vi "Arcade Drive.vi"(0 "Ref In":T1, 7 "X":dbl, 9 "Y":dbl) -> ()   [LabVIEW 2013]
uses:
  Arcade Drive Ref.ctl
  <vilib>/Rock Robotics/WPI/MotorControl/WPI_MotorControlDeviceRef.ctl
  <vilib>/Rock Robotics/SystemInterfaces/Typedef/FPGA_TypedefDigitalModule.ctl
  <vilib>/Rock Robotics/SystemInterfaces/DIO/FPGA_DIOPWMChannel.ctl
  <vilib>/Rock Robotics/WPI/PWM/WPI_PWMDeadband.ctl
  <vilib>/Rock Robotics/WPI/CAN/Jaguar/SubVIs/WPI_CANJaguar_ControlMode.ctl
  <vilib>/Rock Robotics/WPI/PWM/WPI_PWMTransform_ConPane.ctl
  Robot Global Data.vi
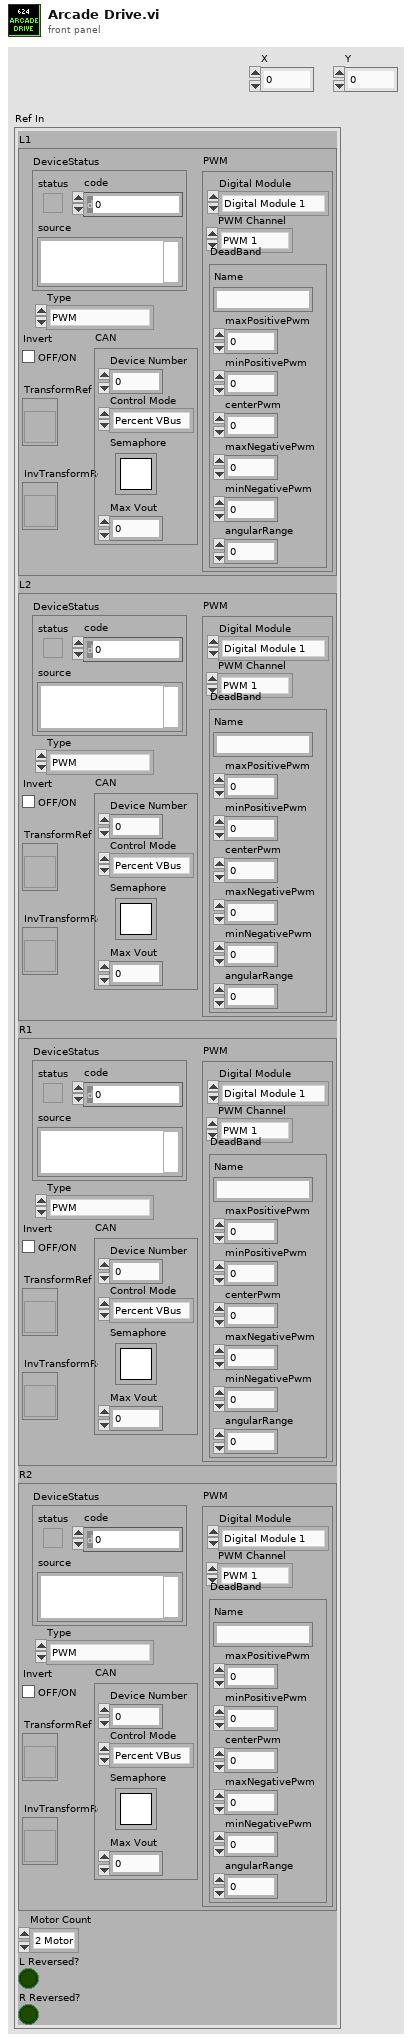
[diagram p1: front panel]
types:
  T1 = typedef "Arcade Drive Ref.ctl" = cluster{"L1":T2, "L2":T2, "R1":T2, "R2":T2, "Motor Count":enum16{"2 Motor", "4 Motor"}, "L Reversed?":bool, "R Reversed?":bool}
  T2 = typedef "WPI_MotorControlDeviceRef.ctl" = cluster{"DeviceStatus":errorcluster, "Type":enum16{"PWM", "CAN"}, "PWM":cluster{"Digital Module":T3, "PWM Channel":T4, "DeadBand":T5}, "CAN":cluster{"Device Number":u8, "Control Mode":T6, "Semaphore":T7, "Max Vout":dbl}, "Invert":bool, "TransformRef":T8, "InvTransformRef":T8}
  T3 = typedef "FPGA_TypedefDigitalModule.ctl" = enum16{"Digital Module 1", "Digital Module 2"}
  T4 = typedef "FPGA_DIOPWMChannel.ctl" = enum8{"PWM 1", "PWM 2", "PWM 3", "PWM 4", "PWM 5", "PWM 6", "PWM 7", "PWM 8", "PWM 9", "PWM 10", "Invalid"}
  T5 = typedef "WPI_PWMDeadband.ctl" = cluster{"Name":string, "maxPositivePwm":i32, "minPositivePwm":i32, "centerPwm":i32, "maxNegativePwm":i32, "minNegativePwm":i32, "angularRange":u16}
  T6 = typedef "WPI_CANJaguar_ControlMode.ctl" = enum8{"Percent VBus", "Current", "Speed", "Position", "Voltage"}
  T7 = typedef "Semaphore RefNum" = refnum<k1>
  T8 = typedef "WPI_PWMTransform_ConPane.ctl" = refnum<vi>
  T9 = typedef "Dashboard UDP Packet.ctl" = cluster{"Camera":T10, "Gyro":T11, "Encoder":T12, "Auto Shift":T13, "Auton":T14, "Drive/Ramp X":dbl, "Drive/Ramp Y":dbl, "Drive/Battery Cutoff":dbl, "Pressure/Compressor Min Voltage":dbl, "Pressure/Compressor Delay":dbl, "Controller/Strafe Correction":bool, "Shooter":T15, "Rollers":T16, "Abort":bool, "Finish":bool}
  T10 = typedef "Camera Controls.ctl" = cluster{"Camera/View Angle X":dbl, "Camera/Goal Track Timeout":dbl, "Camera/View Angle Y":dbl, "Camera/Goal Exposure":dbl, "Camera/Vision Receive Timeout":dbl, "Camera/Offset 1":dbl, "Camera/Offset 2":dbl}
  T11 = typedef "Gyro Controls.ctl" = cluster{"Gyro/Steer Close PID P":dbl, "Gyro/Steer Close PID I":dbl, "Gyro/Steer Close PID D":dbl, "Gyro/Steer Close PID min":dbl, "Gyro/Steer Close PID max":dbl, "Gyro/Steer PID P":dbl, "Gyro/Steer PID I":dbl, "Gyro/Steer PID D":dbl, "Gyro/Steer PID min":dbl, "Gyro/Angle Tolerance":dbl, "Gyro/Steer PID max":dbl, "Gyro/Steer Closeness Threshold":dbl}
  T12 = typedef "Encoder Controls.ctl" = cluster{"Encoders/Reset":bool, "Encoders/Omni Constant":dbl, "Encoders/Omni Tick Constant":dbl, "Encoders/Left Constant":dbl, "Encoders/Right Constant":dbl, "Encoders/Right Tick Constant":dbl}
  T13 = typedef "Auto Shift Controls.ctl" = cluster{"AutoShift/Upshift Throttle Accel":dbl, "AutoShift/Speed Threshold":dbl, "AutoShift/Upshift Throttle":dbl, "AutoShift/Upshift Accel":dbl, "AutoShift/Downshift Accel":dbl, "AutoShift/Downshift Throttle":dbl, "AutoShift/Delay":dbl, "AutoShift/Enabled":bool}
  T14 = typedef "Auton Controls.ctl" = cluster{"Auton/Left Shoot X-Coord":dbl, "Auton/Right Shoot X-Coord":dbl, "DistDrive/Distance Stop Threshold":dbl, "DistDrive/Max Stop Speed":dbl, "Auton/Back Piston Time":dbl, "Auton/Manual Hot":bool, "Auton/Manual Hot Right":bool, "Auton/X Distance PID max":dbl, "Auton/X Distance PID min":dbl, "Auton/X Distance PID P":dbl, "Auton/X Distance PID I":dbl, "Auton/X Distance PID D":dbl, "Auton/Y Distance PID max":dbl, "Auton/Y Distance PID min":dbl, "Auton/Y Distance PID P":dbl, "Auton/Y Distance PID I":dbl, "Auton/Y Distance PID D":dbl}
  T15 = typedef "Shooter Controls.ctl" = cluster{"Shooter/Reset Time":dbl, "Shooter/Release Delay":dbl, "Shooter/Pressure Steady Time":dbl, "Shooter/Misfire Delay":dbl, "Shooter/Ball Settle Time":dbl, "Shooter/Line IR Delay":dbl, "Pressure/Upper PSI Time":dbl, "Pressure/Lower PSI Time":dbl, "Shooter/Punch Delay":dbl, "Shooter/Target Pressure":dbl, "Pressure/Line B":dbl, "Pressure/Line M":dbl, "Pressure/Shooter M":dbl, "Pressure/Shooter B":dbl}
  T16 = typedef "Roller Controls.ctl" = cluster{"Roller/Load IRs Verify Time":dbl, "Roller/Center IR Latch Time":dbl, "Roller/Speed Front":dbl, "Roller/Speed Back":dbl, "Roller/Entry Timeout":dbl, "Roller/To Center Timeout":dbl, "Roller/Sustain Time":dbl, "Roller/Verify Center Time":dbl}
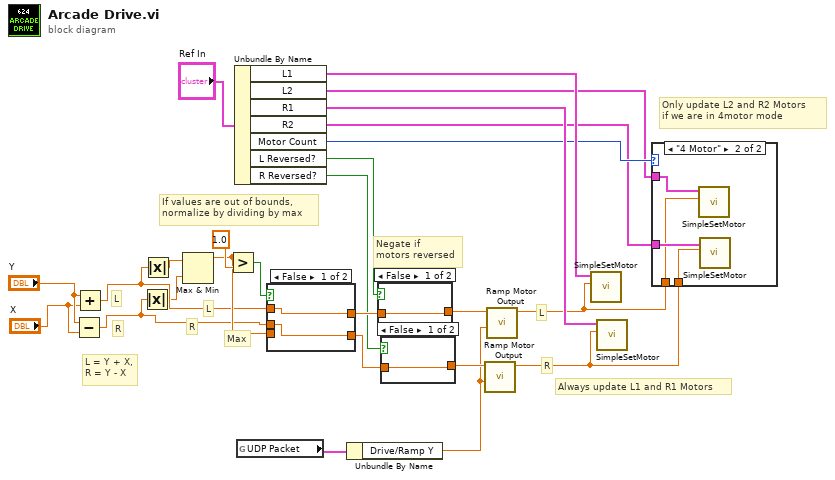
[diagram p0: block diagram]
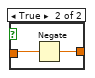
[diagram p3: hidden frame]
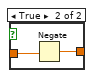
[diagram p4: hidden frame]
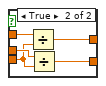
[diagram p5: hidden frame]
diagram:
  # "L = Y + X,\nR = Y - X"
  # "Always update L1 and R1 Motors"
  # "Only update L2 and R2 Motors \nif we are in 4motor mode"
  # "Negate if\nmotors reversed"
  # "R"
  # "L"
  # "R"
  # "L"
  # "Max"
  # "If values are out of bounds,\nnormalize by dividing by max"
  # "R"
  # "L"
  n1 = Subtract(x="Y", y="X") -> (x-y=w7:dbl)
  n2 = Add(x="Y", y="X") -> (x+y=w9:dbl)
  n3 = Absolute Value(x=w7) -> (abs(x)=w8:dbl)
  n4 = Absolute Value(x=w9) -> (abs(x)=w21:dbl)
  n5 = Max & Min(x=w21, y=w8) -> (max(x,y)=w20:dbl)  [unwired: 1 out]
  n6 = Greater?(x=w20, y=1.0) -> (0:w22:bool)
  n7 = Unbundle By Name("Ref In") -> ("L1"=w15:T2, "L2"=w12:T2, "R1"=w14:T2, "R2"=w11:T2, "Motor Count"=w13:enum16{"2 Motor", "4 Motor"}, "L Reversed?"=w19:bool, "R Reversed?"=w17:bool)
  n8 = global read "Robot Global Data.vi" "UDP Packet"() -> (w2:T9)
  n9 = case shown="False" w22 {
    tunnel: w9 -> [w27 w32]
    tunnel: w7 -> [w26 w31]
    tunnel: w20 -> [_ w30]
    tunnel: [w27 w29] -> w18
    tunnel: [w26 w28] -> w16
    frame False {
    }
    frame True {
      n10 = Divide(x=w32, y=w30) -> (x/y=w29:dbl)
      n11 = Divide(x=w31, y=w30) -> (x/y=w28:dbl)
    }
  }
  n12 = Unbundle By Name(w2) -> ("Drive/Ramp Y"=w1:dbl)
  n13 = case shown="False" w19 {
    tunnel: w18 -> [w33 w35]
    tunnel: [w33 w34] -> w4
    frame False {
    }
    frame True {
      n14 = Negate(x=w35) -> (-x=w34:dbl)
    }
  }
  n15 = case shown="False" w17 {
    tunnel: [w36 w38] -> w6
    tunnel: w16 -> [w36 w37]
    frame False {
    }
    frame True {
      n16 = Negate(x=w37) -> (-x=w38:dbl)
    }
  }
  n17 = call "Ramp Motor Output.vi"("Ramp Time"=w1, "Input"=w6) -> ("Output"=w5:dbl)  [unwired: 9 in]
  n18 = call "Ramp Motor Output.vi"("Ramp Time"=w1, "Input"=w4) -> ("Output"=w3:dbl)  [unwired: 9 in]
  n19 = call "SimpleSetMotor.vi"("Output"=w3, "MotorControlDevRef"=w15) -> ()  [unwired: 8 in, 2 out]
  n20 = call "SimpleSetMotor.vi"("Output"=w5, "MotorControlDevRef"=w14) -> ()  [unwired: 8 in, 2 out]
  n21 = case shown="\"4 Motor\"" w13 {
    tunnel: w12 -> [_ w42]
    tunnel: w11 -> [_ w41]
    tunnel: w3 -> [_ w40]
    tunnel: w5 -> [_ w39]
    frame "2 Motor", Default {
    }
    frame "4 Motor" {
      n22 = call "SimpleSetMotor.vi"("Output"=w40, "MotorControlDevRef"=w42) -> ()  [unwired: 8 in, 2 out]
      n23 = call "SimpleSetMotor.vi"("Output"=w39, "MotorControlDevRef"=w41) -> ()  [unwired: 8 in, 2 out]
    }
  }
